vi "SPL meter.vi"() -> ()   [LabVIEW 2018]
panel:
  in  "Off":bool
  in  "Start/Stop":bool
  in  "Filename":path=path "Please enter a file path..."
  in  "Open":bool
  in  "Fast/Slow":bool caption="Blank Button"
  out "Sound Level":bool
  out "Meter":dbl(knob) scale=30.0..130.0
  out "Waveform Chart":waveform(dbl)(graph)
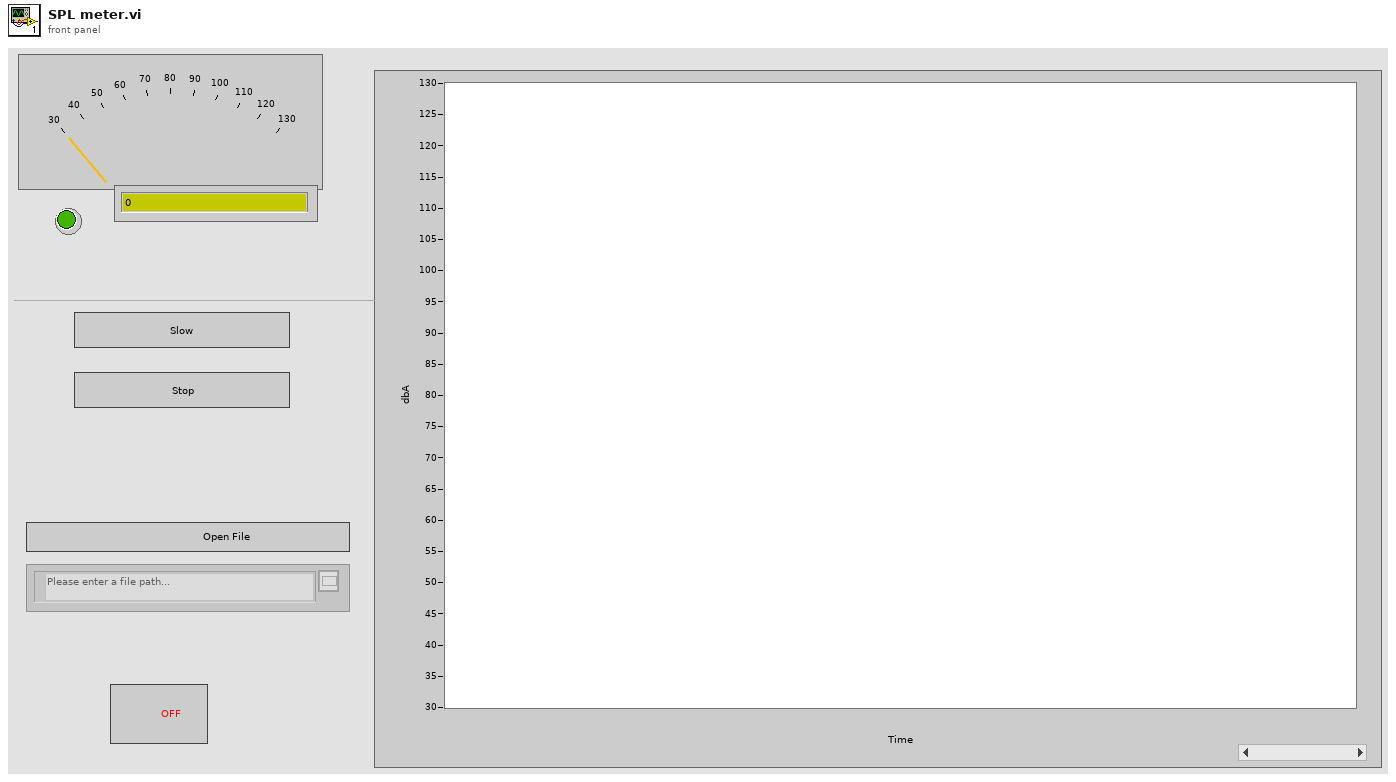
[diagram p1: front panel]
types:
  T1 = enum8{"Enabled", "Disabled", "Disabled and Grayed Out"}
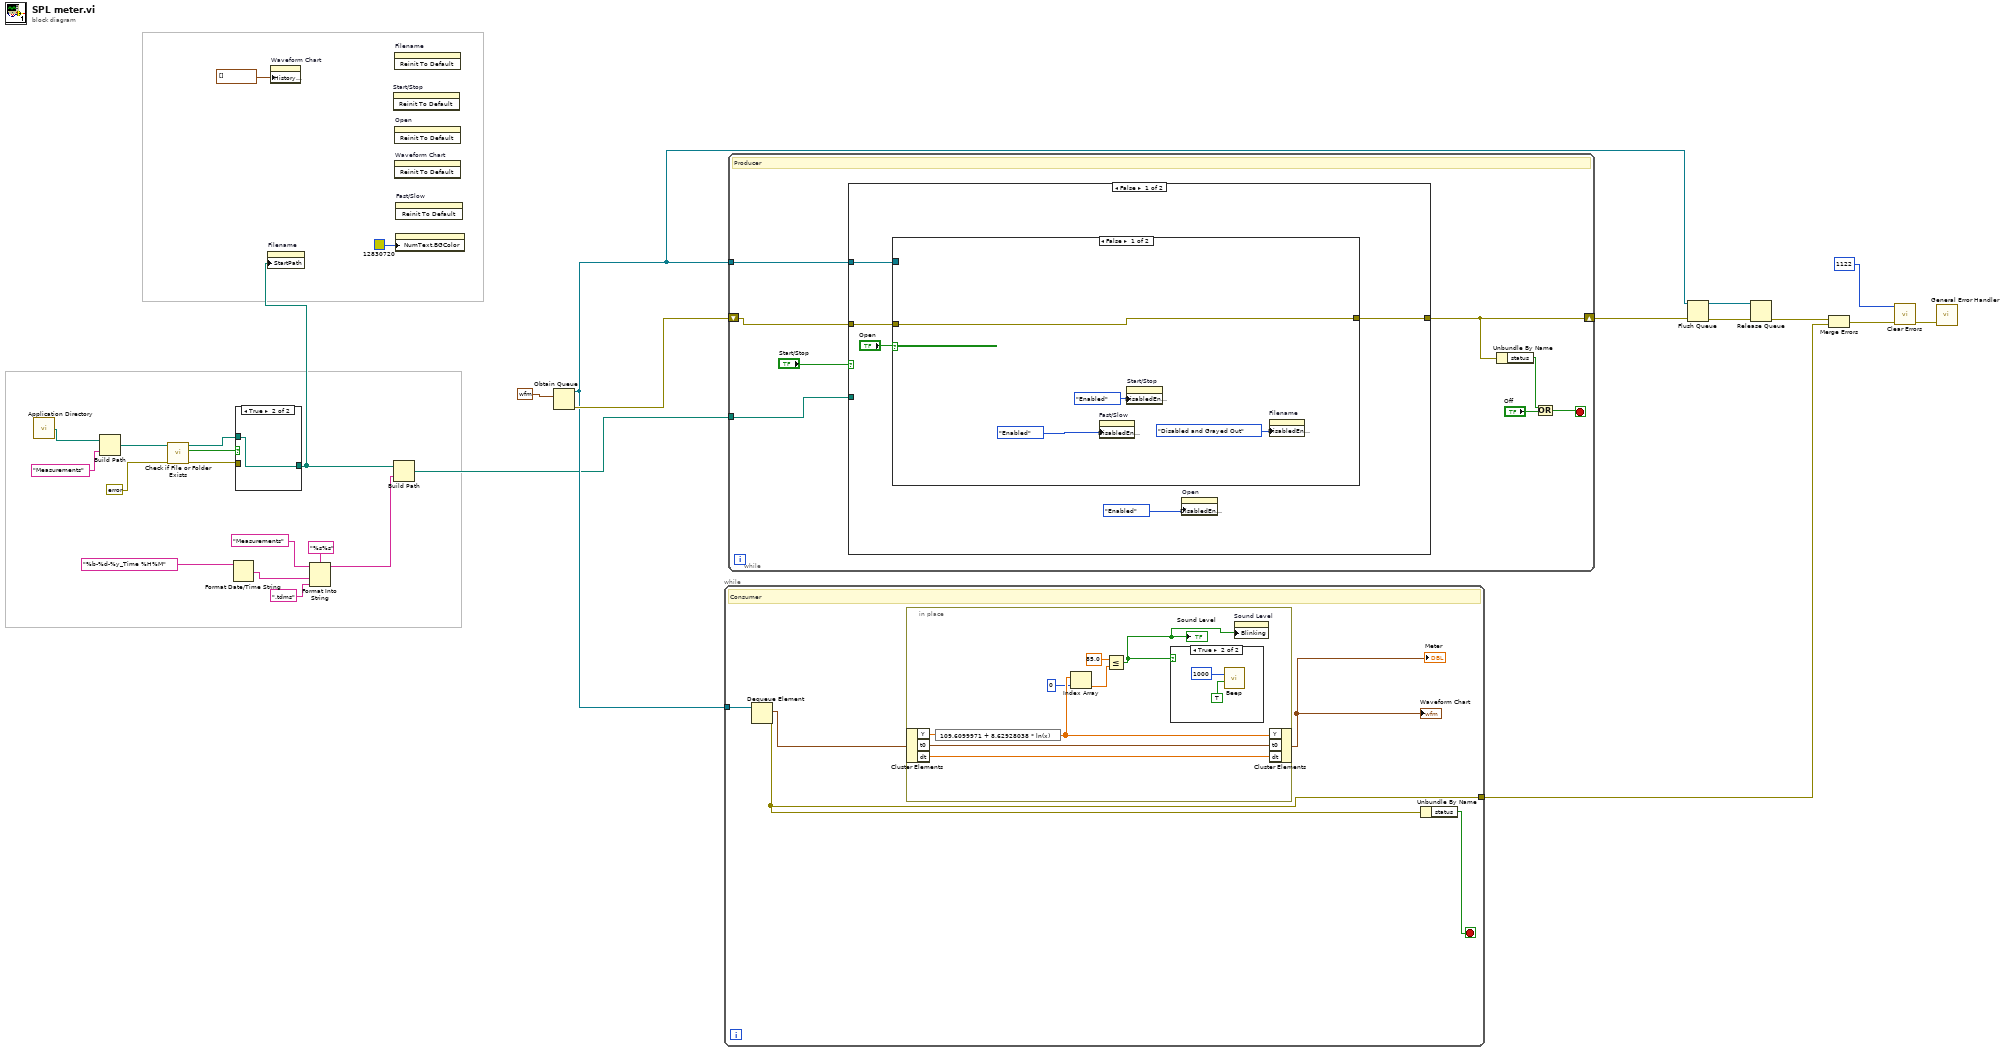
[diagram p0: block diagram]
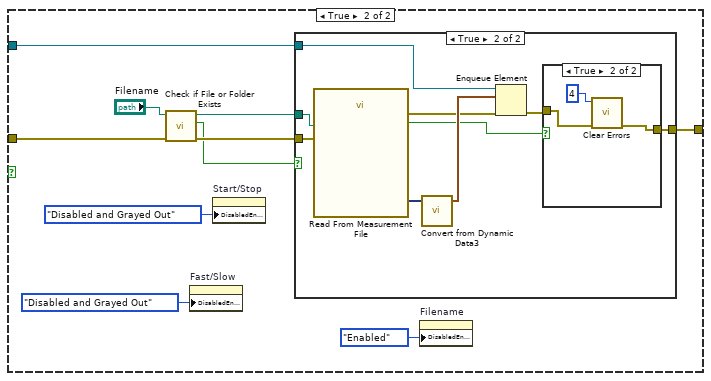
[diagram p3: hidden frame]
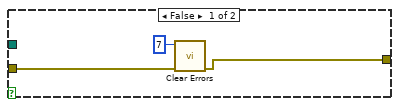
[diagram p4: hidden frame]
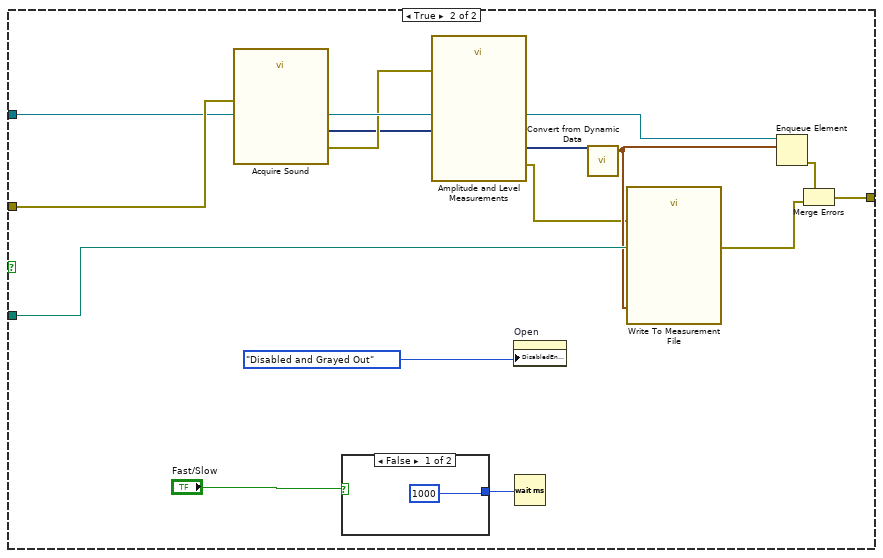
[diagram p6: hidden frame]
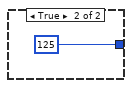
[diagram p7: hidden frame]
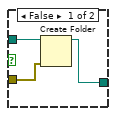
[diagram p8: hidden frame]
diagram:
  n1 = call <vilib>:"Application Directory.vi"() -> ("Application Directory"=w28:path)
  n2 = Build Path(base path=w28, name or relative path="Measurements") -> (appended path=w20:path)
  n3 = call <vilib>:"Check if File or Folder Exists.vi"("error in (no error)"=errorcluster {"status"=FALSE, "code"=0, "source"=""} ("error in"), "path"=w20) -> ("error out"=w16:errorcluster, "file or folder exists?"=w18:bool, "dup path"=w17:path)  [unwired: 7 in]
  n4 = Format Date/Time String(time format string (%c)="%b-%d-%y_Time %H%M") -> (date/time string=w23:string)  [unwired: 2 in]
  n5 = case shown="True" w18 {
    tunnel: [w31 w32] -> w1
    tunnel: w17 -> [w30 w32]
    tunnel: w16 -> [w29 _]
    frame False {
      n6 = Create Folder(path (use dialog)=w30, error in=w29) -> (created path=w31:path)  [unwired: 1 in, 2 out]
    }
    frame True {
    }
  }
  n7 = property on="Filename" class="Path"("StartPath"=w1) -> ()  [unwired: 2 in, 2 out]
  n8 = property on="Waveform Chart" class="WFChart (strict)"("History Data"=waveform(dbl)[] []) -> ()  [unwired: 2 in, 2 out]
  n9 = Format Into String(format string="%s%s", initial string="Measurements", w23, ".tdms" ("input 2")) -> (resulting string=w21:string)  [unwired: 1 in, 1 out]
  n10 = invoke on="Start/Stop" class="Bool (strict)" method="Reinit To Default"() -> ()  [unwired: 3 in, 3 out]
  n11 = Build Path(base path=w1, name or relative path=w21) -> (appended path=w4:path)
  n12 = invoke on="Filename" class="Path" method="Reinit To Default"() -> ()  [unwired: 3 in, 3 out]
  n13 = invoke on="Open" class="Bool (strict)" method="Reinit To Default"() -> ()  [unwired: 3 in, 3 out]
  n14 = invoke on="Waveform Chart" class="WFChart (strict)" method="Reinit To Default"() -> ()  [unwired: 3 in, 3 out]
  n15 = property class="DigNum (strict)"("NumText.BGColor"=u32 12830720) -> ()  [unwired: 2 in, 2 out]
  n16 = invoke on="Fast/Slow" class="Bool (strict)" method="Reinit To Default"() -> ()  [unwired: 3 in, 3 out]
  n17 = Obtain Queue(element data type=waveform(dbl) {"t0"=timestamp(0 s since 1904-01-01), "dt"=1.0, "Y"=[]} ("waveform")) -> (queue out=w7:refnum<queue>, error out=w14:errorcluster)  [unwired: 4 in, 1 out]
  n18 = while {
    tunnel: [w35] -> w13
    tunnel: w7 -> [w37]
    stop <- w34 stop-if-true
    # "Consumer"
    n19 = Dequeue Element(queue=w37) -> (element=w36:waveform(dbl), error out=w35:errorcluster)  [unwired: 2 in, 2 out]
    n20 = in-place {
      n21 = in-place-cluster #1(w36) -> ("Y"=w43:dbl[], "t0"=w45:timestamp, "dt"=w44:dbl)
      n22 = expression code="109.6099971 + 8.62928038 * ln(x)"(w43) -> (w42:dbl[])
      n23 = Index Array(array=w42, index=0) -> (element=w40:dbl)
      n24 = Less Or Equal?(x=85.0, y=w40) -> (x <= y?=w38:bool)
      "Sound Level" <- w38
      n25 = case shown="True" w38 {
        frame False {
        }
        frame True {
          n26 = call <vilib>:"Beep.vi"("use system alert? (T)"=TRUE, "duration (msec)"=u32 1000) -> ()  [unwired: 10 in]
        }
      }
      n27 = property on="Sound Level" class="Bool (strict)"("Blinking"=w38) -> ()  [unwired: 2 in, 2 out]
      n28 = in-place-cluster #1("Y"=w42, "t0"=w45, "dt"=w44) -> (→"Waveform Chart" →"Meter":waveform(dbl))
    }
    n29 = Unbundle By Name(w35) -> ("status"=w34:bool)
  }
  n30 = while "Producer Loop" {
    shift-right: [w49] -> w6
    shift-left: w14 -> [w55]
    tunnel: w7 -> [w54]
    tunnel: w4 -> [w53]
    stop <- w48 stop-if-true
    # "Producer"
    n31 = case shown="False" "Start/Stop" {
      tunnel: w55 -> [w59 w104]
      tunnel: w54 -> [w58 w103]
      tunnel: w53 -> [_ w102]
      tunnel: [w56 w94] -> w49
      frame False {
        n32 = case shown="False" "Open" {
          tunnel: w59 -> [w64 w71]
          tunnel: w58 -> [_ w74]
          tunnel: [w64 w73] -> w56
          frame False {
            n33 = property on="Fast/Slow" class="Bool (strict)"("DisabledEnum"=T1."Enabled" ("Disabled")) -> ()  [unwired: 2 in, 2 out]
            n34 = property on="Start/Stop" class="Bool (strict)"("DisabledEnum"=T1."Enabled" ("Disabled")) -> ()  [unwired: 2 in, 2 out]
            n35 = property on="Filename" class="Path"("DisabledEnum"=T1."Disabled and Grayed Out" ("Disabled")) -> ()  [unwired: 2 in, 2 out]
          }
          frame True {
            n36 = call <vilib>:"Check if File or Folder Exists.vi"("error in (no error)"=w71, "path"="Filename") -> ("error out"=w69:errorcluster, "file or folder exists?"=w68:bool, "dup path"=w70:path)  [unwired: 7 in]
            n37 = property on="Fast/Slow" class="Bool (strict)"("DisabledEnum"=T1."Disabled and Grayed Out" ("Disabled")) -> ()  [unwired: 2 in, 2 out]
            n38 = property on="Start/Stop" class="Bool (strict)"("DisabledEnum"=T1."Disabled and Grayed Out" ("Disabled")) -> ()  [unwired: 2 in, 2 out]
            n39 = case shown="True" w68 {
              tunnel: w74 -> [_ w86]
              tunnel: [w75 w85] -> w73
              tunnel: w70 -> [_ w79]
              tunnel: w69 -> [w77 w78]
              frame False {
                n40 = call <vilib>:"Clear Errors.vi"("error in (no error)"=w77, "specific error code to clear (0: all)"=7) -> ("error out"=w75:errorcluster)  [unwired: 4 in, 1 out]
              }
              frame True {
                n41 = call "Read From Measurement File"("error in (no error)"=w78, "Filename"=w79) -> ("error out"=w80:errorcluster, "Signals"=w83:dynamicdata, "EOF?"=w82:bool)  [unwired: 4 in, 3 out]
                n42 = call "Convert from Dynamic Data3"("Dynamic Data Type"=w83) -> ("Waveform"=w84:waveform(dbl))  [unwired: 3 in]
                n43 = Enqueue Element(queue=w86, element=w84, error in (no error)=w80) -> (error out=w81:errorcluster)  [unwired: 1 in, 2 out]
                n44 = case shown="True" w82 {
                  tunnel: [w87 w90] -> w85
                  tunnel: w81 -> [w87 w88]
                  frame False {
                  }
                  frame True {
                    n45 = call <vilib>:"Clear Errors.vi"("error in (no error)"=w88, "specific error code to clear (0: all)"=4) -> ("error out"=w90:errorcluster)  [unwired: 4 in, 1 out]
                  }
                }
              }
            }
            n46 = property on="Filename" class="Path"("DisabledEnum"=T1."Enabled" ("Disabled")) -> ()  [unwired: 2 in, 2 out]
          }
        }
        n47 = property on="Open" class="Bool (strict)"("DisabledEnum"=T1."Enabled" ("Disabled")) -> ()  [unwired: 2 in, 2 out]
      }
      frame True {
        n48 = call "Acquire Sound"("error in (no error)"=w104) -> ("Data"=w100:dynamicdata, "error out"=w101:errorcluster)  [unwired: 17 in]
        n49 = case shown="False" "Fast/Slow" {
          tunnel: [1000 u32 125 ("milliseconds to wait")] -> w92
          frame False {
          }
          frame True {
          }
        }
        n50 = call "Amplitude and Level Measurements"("Signals"=w100, "error in (no error)"=w101) -> ("RMS"=w99:dynamicdata, "error out"=w97:errorcluster)  [unwired: 12 in]
        n51 = property on="Open" class="Bool (strict)"("DisabledEnum"=T1."Disabled and Grayed Out" ("Disabled")) -> ()  [unwired: 2 in, 2 out]
        n52 = Wait (ms)(milliseconds to wait=w92) -> ()  [unwired: 1 out]
        n53 = call "Convert from Dynamic Data"("Dynamic Data Type"=w99) -> ("Waveform"=w98:waveform(dbl))  [unwired: 3 in]
        n54 = call "Write To Measurement File"("Signals"=w98, "error in (no error)"=w97, "Filename"=w102) -> ("error out"=w95:errorcluster)  [unwired: 14 in, 2 out]
        n55 = Enqueue Element(queue=w103, element=w98) -> (error out=w96:errorcluster)  [unwired: 2 in, 2 out]
        n56 = Merge Errors(w96, w95) -> (w94:errorcluster)
      }
    }
    n57 = Unbundle By Name(w49) -> ("status"=w50:bool)
    n58 = Or(x=w50, y="Off") -> (x .or. y?=w48:bool)
  }
  n59 = Flush Queue(queue=w7, error in (no error)=w6) -> (queue out=w8:refnum<queue>, error out=w5:errorcluster)  [unwired: 1 out]
  n60 = Release Queue(queue=w8, error in (no error)=w5) -> (error out=w11:errorcluster)  [unwired: 1 in, 2 out]
  n61 = Merge Errors(w11, w13) -> (w10:errorcluster)
  n62 = call <vilib>:"Clear Errors.vi"("error in (no error)"=w10, "specific error code to clear (0: all)"=1122) -> ("error out"=w12:errorcluster)  [unwired: 4 in, 1 out]
  n63 = call <vilib>:"General Error Handler.vi"("error in (no error)"=w12) -> ()  [unwired: 10 in, 5 out]
